vi "Run Tx - Loop Delay.vi"(7 "Delay (ms)":u32, 8 "error in (no error)":errorcluster) -> (0 "error out":errorcluster)   [LabVIEW 2021, in "UDP-Custom-Device Engine.lvlib"]
uses:
  UDP-Custom-Device Engine.lvlib
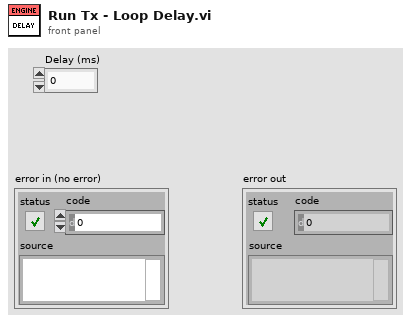
[diagram p1: front panel]
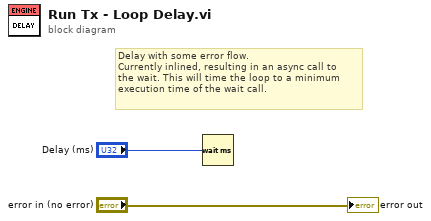
[diagram p0: block diagram]
diagram:
  # "Delay with some error flow.\nCurrently inlined, resulting in an async call to\nthe wait. This will time the loop to a minimum\nexecution time of the wait call."
  n1 = Wait (ms)(milliseconds to wait="Delay (ms)") -> ()  [unwired: 1 out]
  "error out" <- "error in (no error)"
